vi "mupDefineVar.vi"(8 "error in (no error)":errorcluster, 9 "initValue":dbl, 10 "varName":string, 11 "hParser in":u64) -> (0 "error out":errorcluster, 2 "varAddr":u64, 3 "hParser out":u64)   [LabVIEW 2015, in "mupLib.lvlib"]
doc: "Define a variable and set its initial value.\nThe variable's pointer is returned in varAddr."
uses:
  mupLib.lvlib
  <vilib>/Utility/error.llb/Error Cluster From Error Code.vi
panel:
  # "Define a variable and set its initial value.\nThe variable's pointer is returned in varAddr."
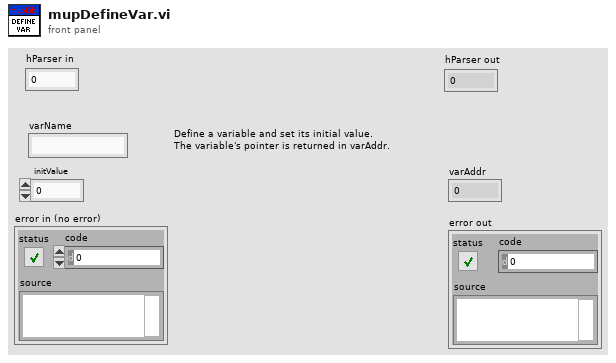
[diagram p1: front panel]
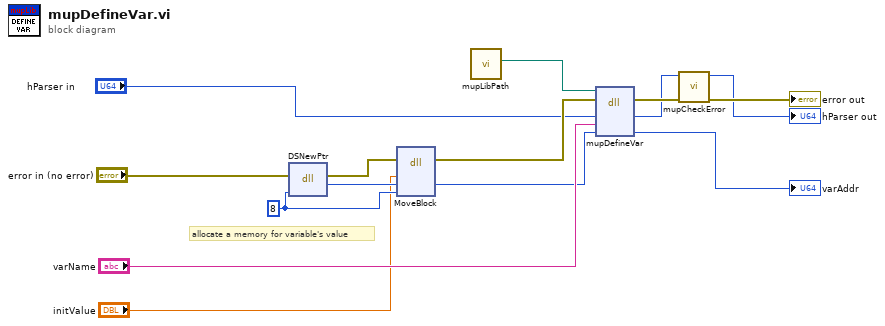
[diagram p0: block diagram]
diagram:
  w14 = 8 ("size")
  # "allocate a memory for variable's value"
  n1 = dll-call lib="LabVIEW" fn="DSNewPtr"(error in="error in (no error)", "size"=w14) -> (error out=w13:errorcluster, "return type"=w15:u64)  [unwired: 3 in, 1 out]
  n2 = dll-call lib="LabVIEW" fn="MoveBlock"(error in=w13, "ps"="initValue", "pd"=w15, "size"=w14) -> (error out=w12:errorcluster, "pd"=w10:u64)  [unwired: 5 in, 1 out]
  n3 = call "mupLibPath.vi"() -> ("libmuparser path"=w2:path)  [unwired: 11 in]
  n4 = dll-call lib="usr/lib/x86_64-linux-gnu/libmuparser.so.2" fn="mupDefineVar"(path in=w2, error in=w12, "hParser"="hParser in", "szName"="varName", "fVar"=w10) -> (error out=w7:errorcluster, "hParser"=w3:u64, "fVar"=→"varAddr":u64)  [unwired: 3 in, 1 out]
  n5 = call "mupCheckError.vi"("error in (no error)"=w7, "hParser in"=w3) -> ("error out"=→"error out":errorcluster, "hParser out"=→"hParser out":u64)  [unwired: 8 in]
